vi "Errors.vi"(9 "Error Codes":u16, 10 "Status":bool, 11 "Error in":cluster{"status":bool, "Codes":u16[]}={"status"=FALSE, "Codes"=[0, 0, 0]}) -> (2 "Status":bool, 3 "Error out":cluster{"status":bool, "Codes":u16[]})   [LabVIEW 2015]
uses:
  Code/Codes Transfer/LabVIEW and LabVIEW FPGA/Globals/Error Index.vi
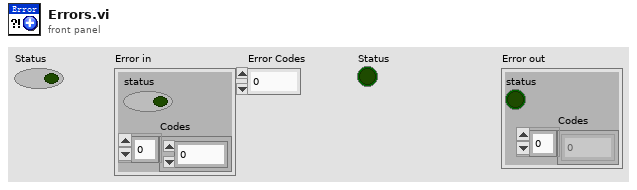
[diagram p1: front panel]
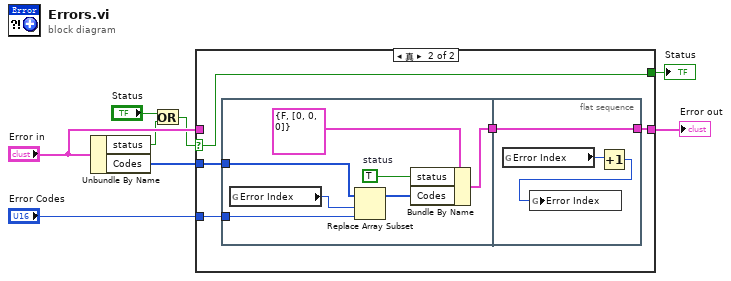
[diagram p0: block diagram]
diagram:
  n1 = Unbundle By Name("Error in") -> ("status"=w3:bool, "Codes"=w8:u16[])
  n2 = Or(x="Status", y=w3) -> (x .or. y?=w2:bool)
  n3 = case shown="真" w2 {
    selector: w2 -> [w9 w11]
    tunnel: w8 -> [_ w15]
    tunnel: "Error Codes" -> [_ w14]
    tunnel: [w10 w12] -> w5
    tunnel: "Error in" -> [w10 _]
    tunnel: [w9 w11] -> w1
    frame False {
    }
    frame True {
      n4 = flat-sequence {
        tunnel: w15 -> [w20]
        tunnel: w14 -> [w18]
        tunnel: [w16] -> w13
        tunnel: w13 -> [w23]
        tunnel: [w23] -> w12
        frame #0 {
          w22 = TRUE  # status
          n5 = global read "Error Index.vi" "Error Index"() -> (w19:enum16{"0", "1", "2"})
          n6 = Replace Array Subset(array=w20, new element=w18, index=w19) -> (w17:u16[])
          n7 = Bundle By Name(cluster=cluster{"status":bool, "Codes":u16[]} {"status"=FALSE, "Codes"=[0, 0, 0]} ("错误输入"), "status"=w22, "Codes"=w17) -> (w16:cluster{"status":bool, "Codes":u16[]})
        }
        frame #1 {
          n8 = global read "Error Index.vi" "Error Index"() -> (w25:enum16{"0", "1", "2"})
          n9 = Increment(x=w25) -> (x+1=w24:enum16{"0", "1", "2"})
          n10 = global write "Error Index.vi" "Error Index"(w24) -> ()
        }
      }
    }
  }
  "Error out" <- w5
  "Status" <- w1
